vi "Read Channels.vi"(8 "error in (no error)":errorcluster, 11 "Pressure Monitor in":refnum<class "Pressure Monitor.lvclass">) -> (0 "error out":errorcluster, 2 "Channels":refnum<class "HK Item.lvclass">[](array[class]), 3 "Pressure Monitor out":refnum<class "Pressure Monitor.lvclass">)   [LabVIEW 2021, in "Pressure Monitor.lvclass"]
uses:
  Pressure Monitor.lvclass
  hk-channel-class/HK Item/HK Item.lvclass
  Pressure Monitor.lvclass/Pressure Monitor.ctl
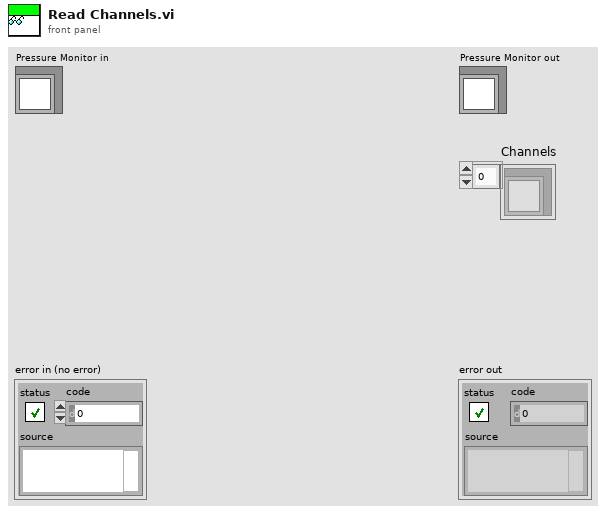
[diagram p1: front panel]
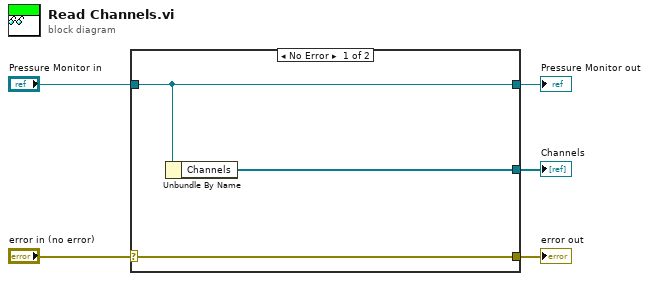
[diagram p0: block diagram]
diagram:
  n1 = case shown="No Error" "error in (no error)" {
    selector: "error in (no error)" -> [w8 w9]
    tunnel: [w8 w9] -> w4
    tunnel: [w7 w10] -> w2
    tunnel: "Pressure Monitor in" -> [w7 w10]
    tunnel: [w6 _] -> w1
    frame No Error {
      n2 = Unbundle By Name(w7) -> ("Channels"=w6:refnum<class "HK Item.lvclass">[])
    }
    frame Error {
    }
  }
  "error out" <- w4
  "Pressure Monitor out" <- w2
  "Channels" <- w1
